vi "Thread@ForeachBreak__Parameter.vi"(1 "ParamterIn":string) -> (0 "ParamterOut":string)   [LabVIEW 2020]
panel:
  in  "Confirm":bool
  in  "IOLogic":string(combo)
  # "Thread@ForeachBreak $IOLogic\nIOLogic Express is:\nIO1 & (IO2 | IO3)\nVar==XXX, !=XXX, >=XXX, <=XXX, >XXX, <XXX\nVar <> XXX~YYY, </>XXX~YYY\nVar==NULL, ==EXIST, ==[],==[;;]\n~IOLogic will inverse Logic"
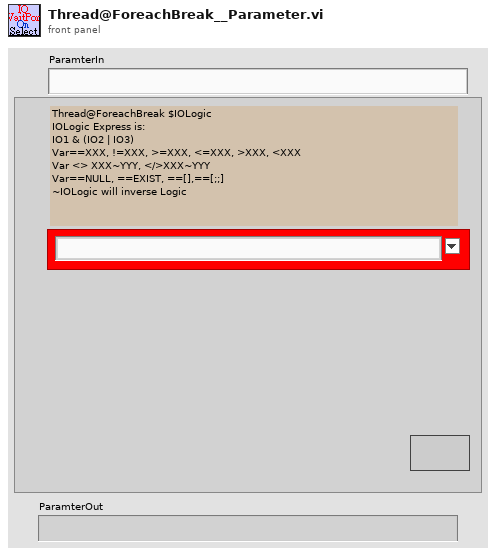
[diagram p1: front panel]
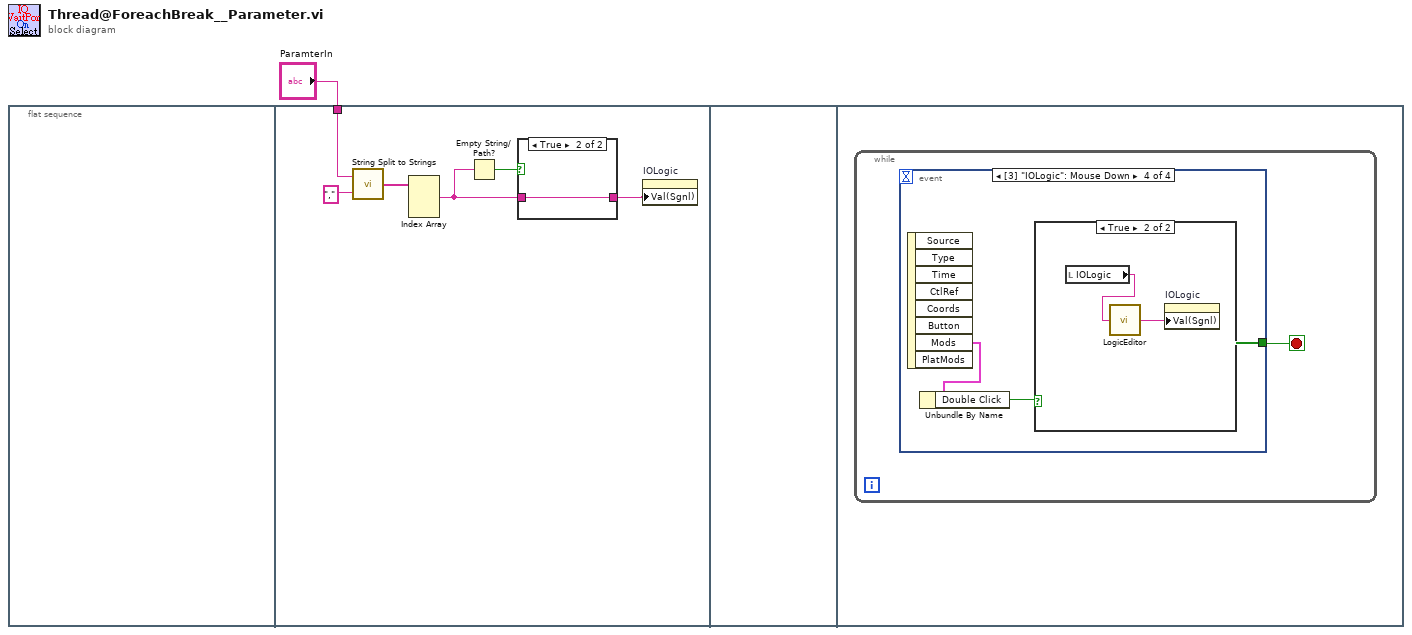
[diagram p0: block diagram]
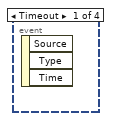
[diagram p3: hidden frame]
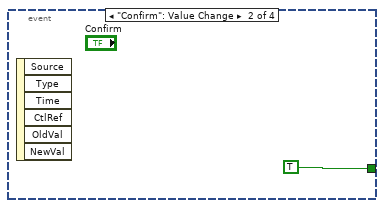
[diagram p4: hidden frame]
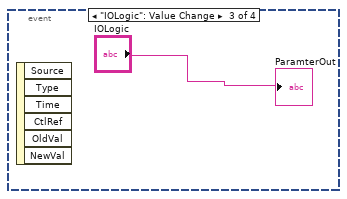
[diagram p5: hidden frame]
diagram:
  n1 = flat-sequence {
    tunnel: "ParamterIn" -> [w6]
    frame #0 {
    }
    frame #1 {
      n2 = call "String Split to Strings.vi"("search string/char (-)"=",", "String"=w6) -> ("Array"=w5:string[])
      n3 = Index Array(array=w5) -> (element #1=w3:string)  [unwired: 3 in, 2 out]
      n4 = Empty String/Path?(string/path=w3) -> (empty?=w4:bool)
      n5 = case shown="True" w4 {
        tunnel: w3 -> [w8 w9]
        tunnel: [w8 w9] -> w2
        frame False {
        }
        frame True {
        }
      }
      n6 = property on="IOLogic" class="CmbBox"("Val(Sgnl)"=w2) -> ()  [unwired: 2 in, 2 out]
    }
    frame #2 {
    }
    frame #3 {
      n7 = while {
        stop <- w10 stop-if-true
        n8 = event shown="[3] \"IOLogic\": Mouse Down" {
          selector: _ -> [_ _ _ _]
          dyn-events: _ -> [_ _ _ _]
          timeout: _ -> [_ _ _ _]
          tunnel: [_ TRUE _ _] -> w10
          event Timeout {
            n9 = event-data() -> ()  [unwired: 1 in, 3 out]
          }
          event "Confirm": Value Change {
            n10 = event-data() -> ()  [unwired: 1 in, 6 out]
          }
          event "IOLogic": Value Change {
            n11 = event-data() -> ()  [unwired: 1 in, 6 out]
            "ParamterOut" <- "IOLogic"
          }
          event "IOLogic": Mouse Down {
            n12 = event-data() -> ("Mods"=w14:cluster{"Double Click":bool, "Menu Key":bool})  [unwired: 1 in, 7 out]
            n13 = Unbundle By Name(w14) -> ("Double Click"=w13:bool)
            n14 = case shown="True" w13 {
              frame False {
              }
              frame True {
                n15 = local read "IOLogic"() -> (w16:string)
                n16 = call "LogicEditor.vi"("Logic Express"=w16) -> ("LogicExpressOut"=w15:string)
                n17 = property on="IOLogic" class="CmbBox"("Val(Sgnl)"=w15) -> ()  [unwired: 2 in, 2 out]
              }
            }
          }
        }
      }
    }
  }
